vi "convert histogram data.vi"(10 "data out":u8[](array[numeric])) -> (1 "count histogram":u32[](array[numeric]), 2 "cycle histogram":u32[](array[numeric]), 4 "detection histogram":u32[](array[numeric]))   [LabVIEW 2017]
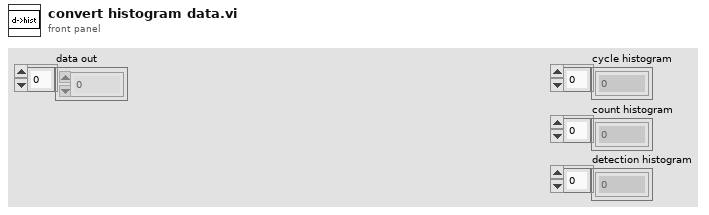
[diagram p1: front panel]
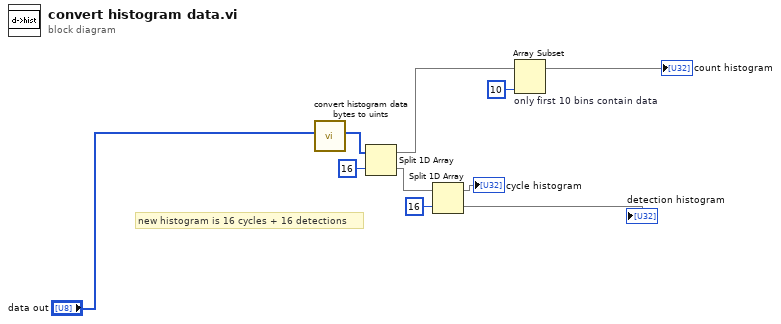
[diagram p0: block diagram]
diagram:
  # "new histogram is 16 cycles + 16 detections"
  n1 = call "convert histogram data bytes to uints.vi"("data out"="data out") -> ("uint data"=w9:u32[])  [unwired: 10 in]
  n2 = Split 1D Array(array=w9, index=16) -> (first subarray=w4:u32[], second subarray=w7:u32[])
  n3 = Split 1D Array(array=w7, index=16) -> (first subarray=→"cycle histogram":u32[], second subarray=→"detection histogram":u32[])
  n4 = Array Subset "only first 10 bins contain data"(array=w4, length=10) -> (→"count histogram":u32[])  [unwired: 1 in]
